vi "FXP_X_minus_Nx_times_ye_singleAxis.vi"(7 "NS":u8=5, 8 "yd_est_x":fxp<+/-,32,5>, 11 "ref(k)_x":fxp<+/-,32,5>) -> (0 "xu_k":fxp<+/-,32,6>, 3 "xerr":T1)   [LabVIEW 2017]
uses:
  typeDefs/x_vec_type.ctl
  <vilib>/Platform/TimedLoop/XDataNode/timing_clust.ctl
  <vilib>/Platform/TimedLoop/XDataNode/nitl_modes.ctl
  <vilib>/Platform/TimedLoop/XDataNode/wakeup.ctl
  typeDefs/x_vec_bram.ctl
  typeDefs/Nx_bram.ctl
  <vilib>/rvi/Emulation/niFpgaSctlEmulationGetInTimedLoop.vi
  <vilib>/rvi/Emulation/niFpgaEmulationReportErrorSimple.vi
  <vilib>/rvi/Emulation/niFpgaGetClockAttributes.vi
  <vilib>/rvi/Emulation/niFpgaCriticalErrorInLSC.vi
  <vilib>/rvi/DataTransferAndStorage/Container/Common/niFpgaContainerExecOnDevCompGetState.vi
  <vilib>/rvi/Emulation/niFpgaEmulationIsFPGAContextNoSignature.vi
  <vilib>/rvi/DataTransferAndStorage/Container/Common/niFpgaContainerGetUniqueNameForEmu.vi
  <vilib>/rvi/Emulation/niFpgaProcessEmulError.vi
  <vilib>/rvi/errors/nirviReportUnexpectedCaseInternalError (U32).vi
  <vilib>/rvi/Memory/Memory_Emulation/niFpgaMemoryEmulationCacheClearOnFirstRun.vi
  <vilib>/rvi/Memory/Memory_Emulation/nirvimemoryEmulationManagerCache_MakeExclusive.vi
  <vilib>/rvi/Memory/Memory_Emulation/niFpgaMemoryEmulationValidateCache.vi
  <vilib>/rvi/Memory/Memory_Emulation/nirvimemoryEmulationManagerCache_InsertValue.vi
  <vilib>/Utility/error.llb/Clear Errors.vi
  <vilib>/rvi/Memory/Memory_Emulation/nirvimemoryEmulationManagerCache_ReleaseExclusive.vi
  <vilib>/rvi/Memory/Memory_Emulation/nirvimemoryEmulationManagerCache_GetValue.vi
  <vilib>/rvi/Memory/Memory_Emulation/nirvimemoryEmulationManagerCache_SetValue.vi
  <vilib>/rvi/Emulation/niFpgaSctlEmulationResourceMgr.vi
  <vilib>/Platform/TimedLoop/XDataNode/XDataNode.xnode
  <vilib>/rvi/FXPMathLib/FxpSub/XNode/nifxpmath_Sub.xnode
  <vilib>/rvi/DataTransferAndStorage/Container/XNode/niFpgaContainer.xnode
  <vilib>/rvi/Memory/Memory_Emulation/niFpgaMemoryEmulationRefIn.vi
  <vilib>/Platform/TimedLoop/XDataNode/XDNodeRunTimeDep.lvlib
  <vilib>/rvi/FXPMathLib/sim/FxpSim.dll
panel:
  # "|x(k)   |    -  |dcg*xss| *(r(k)-x_d(k))\n|x_u(k)|       |dcg      |\n\nx_u:  = x(k-1)\nx_d  = disturbance estimate."
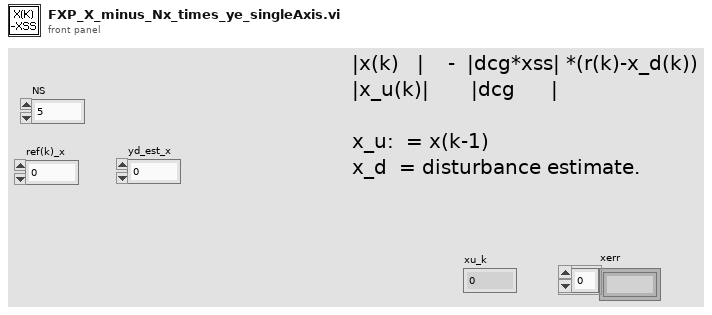
[diagram p1: front panel]
types:
  T1 = typedef "x_vec_type.ctl" = fxp<+/-,32,6>[]
  T2 = typedef "XDNodeRunTimeDep.lvlib/timing_clust.ctl" = cluster{"Expected End [f-1]":u64, "Actual End [f-1]":u64, "Finished Late? [f-1]":bool, "Expected End [i-1]":u64, "Actual End [i-1]":u64, "Finished Late? [i-1]":bool, "Expected Start [i]":u64, "Actual Start [i]":u64, "Expected Start [f]":u64, "Actual Start [f]":u64, "Source Name":string, "Structure Name":string, "Period":i64, "Deadline":i64, "Offset":i64, "Start":i64, "Priority":i32, "Timeout":i32, "Mode":T3, "Wakeup Reason":T4, "Error":errorcluster, "Source Type":string, "Secondary Source Type":string, "Global End Time":u64, "Global Start Time":u64, "Frame Duration":u64, "Iteration Duration":u64, "Assigned CPU":i32, "I/O Scan Engine Mode":u32}
  T3 = typedef "XDNodeRunTimeDep.lvlib/nitl_modes.ctl" = enum32{"No Change", "Process missed periods, maintain original phase", "Discard missed periods, maintain original phase", "Process missed periods, ignore original phase", "Discard missed periods, ignore original phase"}
  T4 = typedef "XDNodeRunTimeDep.lvlib/wakeup.ctl" = enum32{"Normal", "Aborted", "Asynchronous wakeup", "Timing source error", "Timed loop error", "Timeout"}
  T5 = typedef "Nx_bram.ctl" = refnum<k21>
  T6 = typedef "x_vec_bram.ctl" = refnum<k21>
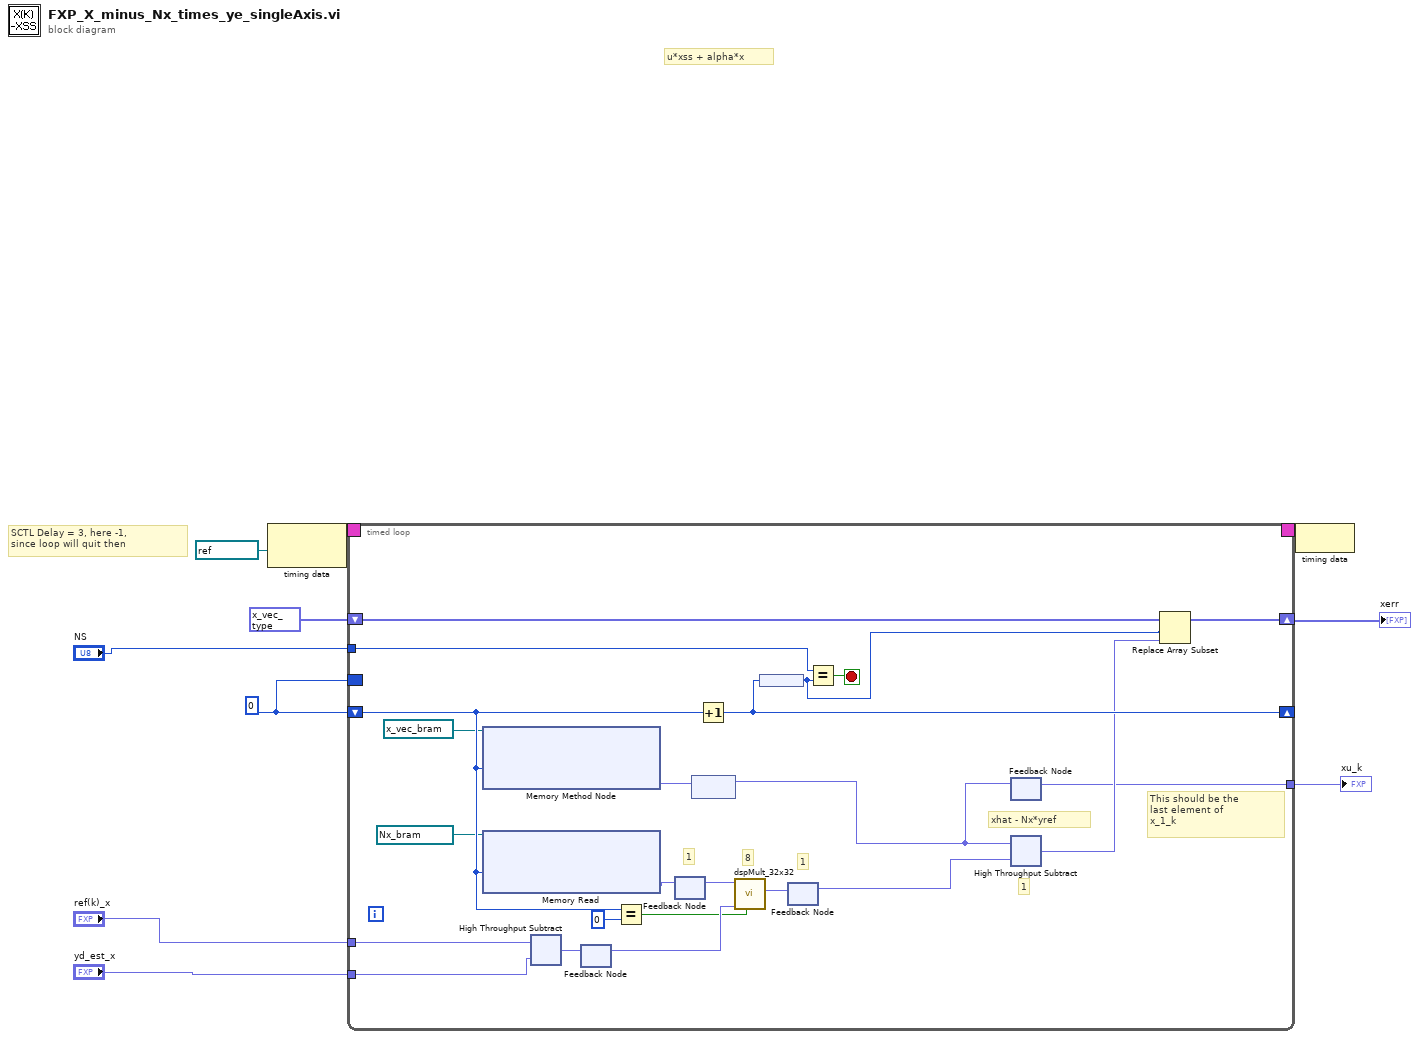
[diagram p0: block diagram]
diagram:
  w6 = u8 0
  # "u*xss + alpha*x"
  # "SCTL Delay = 3, here -1,\nsince loop will quit then"
  n1 = node-c288(refnum<k21> "80MHz" ("Source Name")) -> (w10:T2)
  n2 = timed-loop {
    timing: w10 -> [_]
    timing-out: [_] -> w9
    tunnel: "ref(k)_x" -> [w31]
    tunnel: "yd_est_x" -> [w30]
    shift-right: [w24] -> _
    shift-left: w6 -> [w22]
    tunnel: "NS" -> [w27]
    border: w6 -> [_]
    tunnel: [w16] -> w3
    shift-right: [w19] -> w2
    shift-left: T1 [0.0, 0.0, 0.0, 0.0, 0.0, 0.0, 0.0, 0.0, 0.0, 0.0, 0.0, 0.0, 0.0, 0.0, 0.0, 0.0, 0.0, 0.0, 0.0, 0.0, 0.0, 0.0, 0.0, 0.0, 0.0] ("xerr 2") -> [w18]
    stop <- w33 stop-if-true
    # "This should be the \nlast element of \nx_1_k"
    # "1"
    # "xhat - Nx*yref"
    # "1"
    # "8"
    # "1"
    n3 = xnode ("Memory Method Node")("Address"=w22, "Memory In"=T6 "xk_1_2" ("Memory")) -> ("Data"=w32:fxp<+/-,32,6>)  [unwired: 1 out]
    n4 = xnode ("Memory Read")("Address"=w22, "Memory In"=T5 "Nx_col1" ("Nx")) -> ("Data"=w29:fxp<+/-,32,2>)  [unwired: 1 out]
    n5 = xnode "High Throughput Subtract"("x"=w31, "y"=w30) -> ("x-y"=w28:fxp<+/-,32,5>)
    n6 = feedback #1() -> (w23:fxp<+/-,32,5>)  [unwired: 1 in]
    n7 = feedback-in #1(w28) -> ()
    n8 = Equal?(x=w22, y=u8 0) -> (x = y?=w20:bool)
    n9 = feedback #2() -> (w25:fxp<+/-,32,2>)  [unwired: 1 in]
    n10 = feedback-in #2(w29) -> ()
    n11 = feedback #3() -> (w15:fxp<+/-,32,6>)  [unwired: 1 in]
    n12 = feedback-in #3(w32) -> ()
    n13 = Increment(x=w22) -> (x+1=w24:u8)
    n14 = call "dspMult_32x32.vi"("sclr"=w20, "b"=w23, "a"=w25) -> ("p"=w26:fxp<+/-,64,10>)  [unwired: 8 in]
    n15 = feedback #4() -> (w13:u8)
    n16 = feedback-in #4(w24) -> ()
    n17 = feedback #5() -> (w14:fxp<+/-,64,10>)  [unwired: 1 in]
    n18 = feedback-in #5(w26) -> ()
    n19 = Equal?(x=w27, y=w13) -> (x = y?=w33:bool)
    n20 = feedback #6() -> (w16:fxp<+/-,32,6>)  [unwired: 1 in]
    n21 = feedback-in #6(w15) -> ()
    n22 = xnode "High Throughput Subtract"("x"=w15, "y"=w14) -> ("x-y"=w17:fxp<+/-,32,6>)
    n23 = Replace Array Subset(array=w18, new element=w17, index=w13) -> (w19:T1)
  }
  "xu_k" <- w3
  "xerr" <- w2
  n24 = node-c288(w9) -> ()
